vi "ZLIB Store__ogtk.vi"   [LabVIEW 2016]
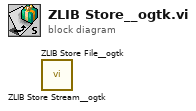
[diagram p0: block diagram]
diagram:
  n1 = call <userlib>:"ZLIB Store Stream__ogtk.vi"() -> ()  [unwired: 10 in, 2 out]
  n2 = call <userlib>:"ZLIB Store File__ogtk.vi"() -> ()  [unwired: 10 in, 2 out]
